vi "HardwareRangeStrings.vi"(8 "error in (no error)":errorcluster, 11 "Pstat IN":refnum<k7>) -> (0 "error out":errorcluster, 2 "Hardware Strings":T1={"I/E Ranges"=[], "First I/E Range"=0, "VchRanges"=[], "IchRanges"=[], "AchRanges"=[], "VchFilters"=[], "IchFilters"=[], "AchFilters"=[], "Family"="", "CA Speeds"=[], "ModelNo"=32} {"ModelNo" items=["PC4300"=32, "PC4750"=33, "PCI4300"=34, "PCI4750"=35, "FAS1"=16, "FC350"=17, "FAS2"=18, "FCI350"=19, "PC5600"=4, "PCI4G300"=36, "PCI4G750"=37, "FCIG350"=21, "REF3000"=5, "REF30K"=6]}, 3 "Pstat OUT":refnum<k7>)   [LabVIEW 2011]
panel:
  out "ModelNo":i32(ring)=32 items=["PC4300"=32, "PC4750"=33, "PCI4300"=34, "PCI4750"=35, "FAS1"=16, "FC350"=17, "FAS2"=18, "FCI350"=19, "PC5600"=4, "PCI4G300"=36, "PCI4G750"=37, "FCIG350"=21, "REF3000"=5, "REF30K"=6]
  out "TestIERange 100":i32
  out "TestIERange 0":i32
  out "CA Speeds":string[](array[string])=["Fast\n", "Normal", "Medium", "Slow"]
  out "Family":string="PC5"
  out "AchFilters":string[](array[string])=["30 mV", "300 mV", "3 V", "12 V"]
  out "IchFilters":string[](array[string])=["30 mV", "300 mV", "3 V", "12 V"]
  out "VchFilters":string[](array[string])=["30 mV", "300 mV", "3 V", "12 V"]
  out "AchRanges":string[](array[string])=["30 mV", "300 mV", "3 V", "12 V"]
  out "IchRanges":string[](array[string])=["30 mV", "300 mV", "3 V", "12 V"]
  out "VchRanges":string[](array[string])=["30 mV", "300 mV", "3 V", "12 V"]
  out "First I/E Range":i32=1
  out "I/E Ranges":string[](array[string])
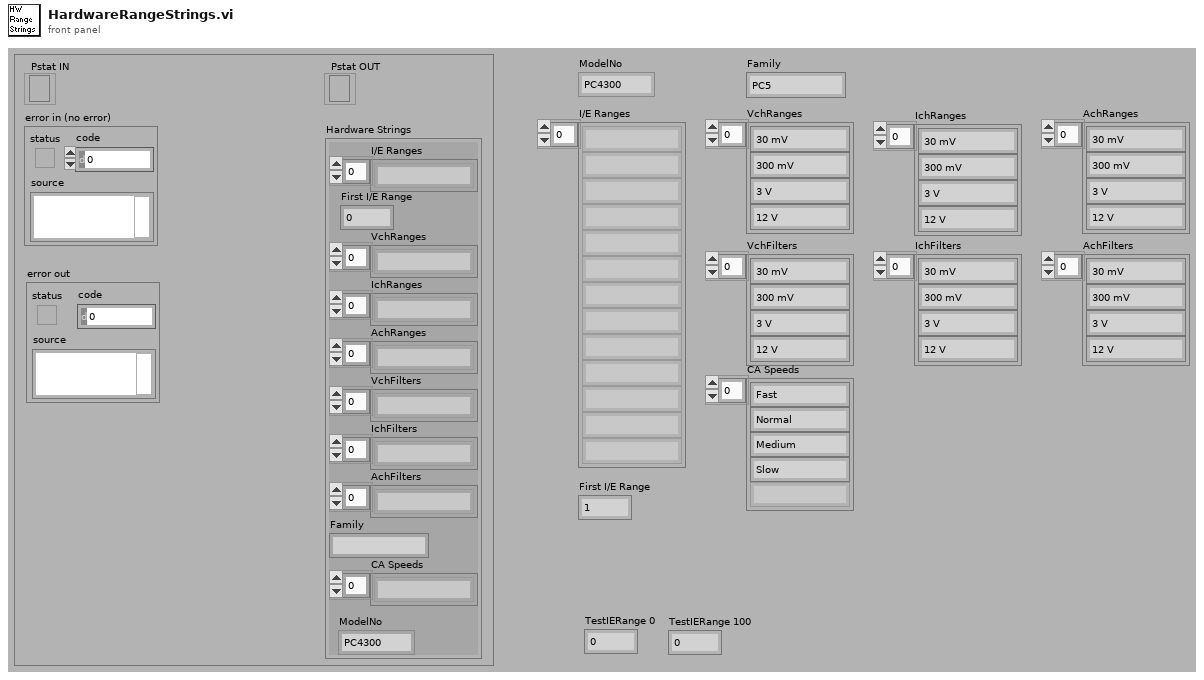
[diagram p1: front panel]
types:
  T1 = cluster{"I/E Ranges":string[], "First I/E Range":i32, "VchRanges":string[], "IchRanges":string[], "AchRanges":string[], "VchFilters":string[], "IchFilters":string[], "AchFilters":string[], "Family":string, "CA Speeds":string[], "ModelNo":i32}
  T2 = cluster{string[], i32, string[], string[], string[], string[], string[], string[], string, string[], "ModelNo":i32}
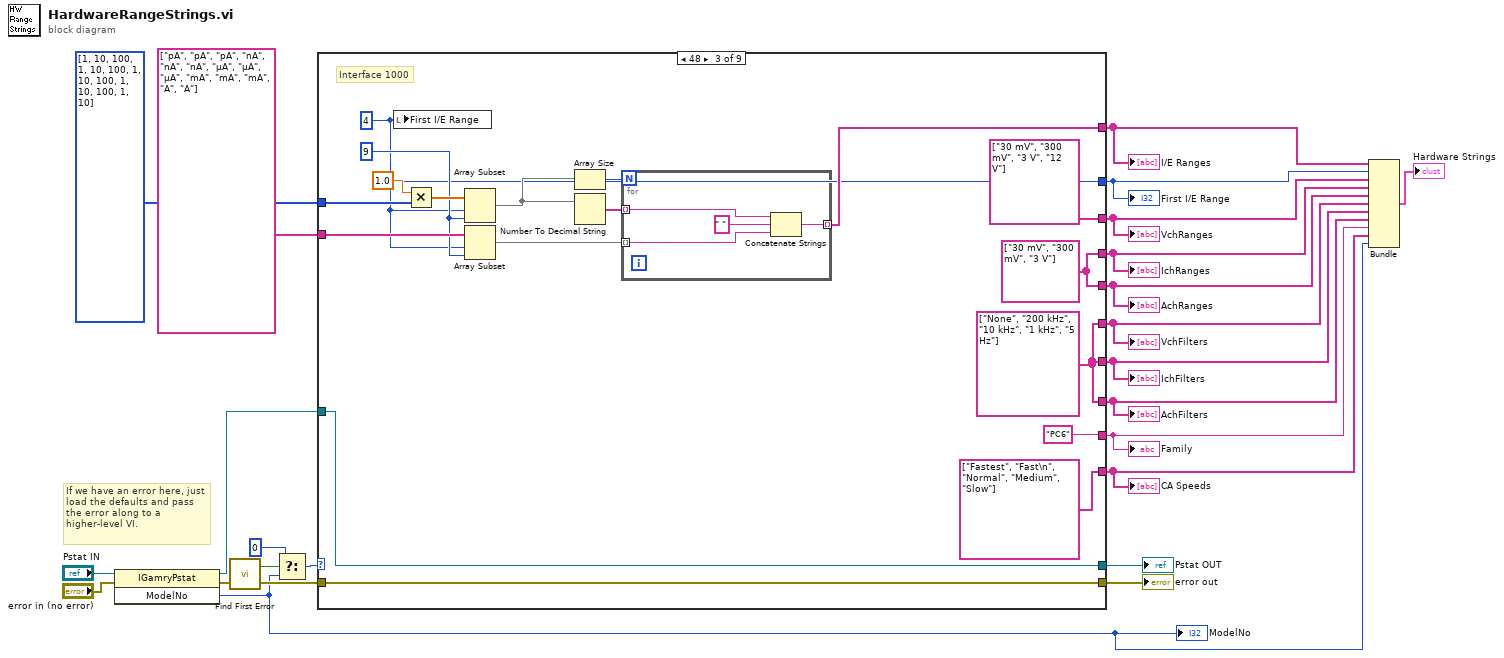
[diagram p0: block diagram]
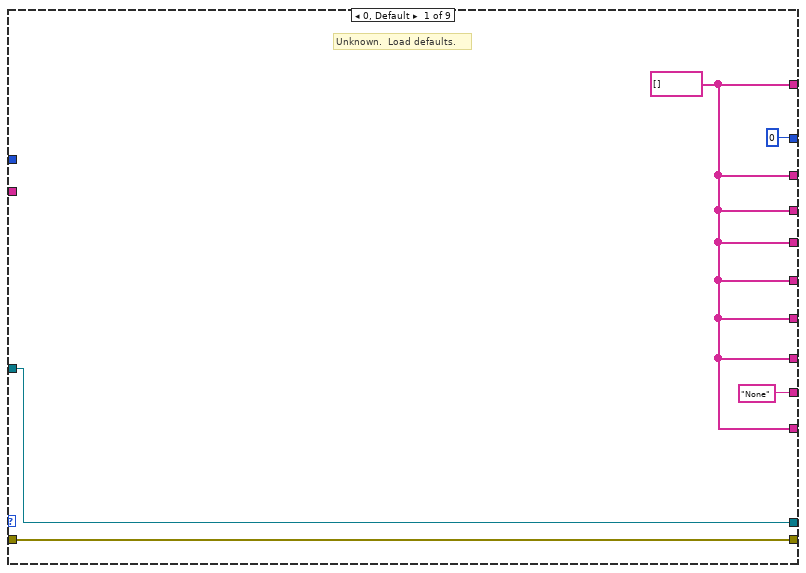
[diagram p2: hidden frame]
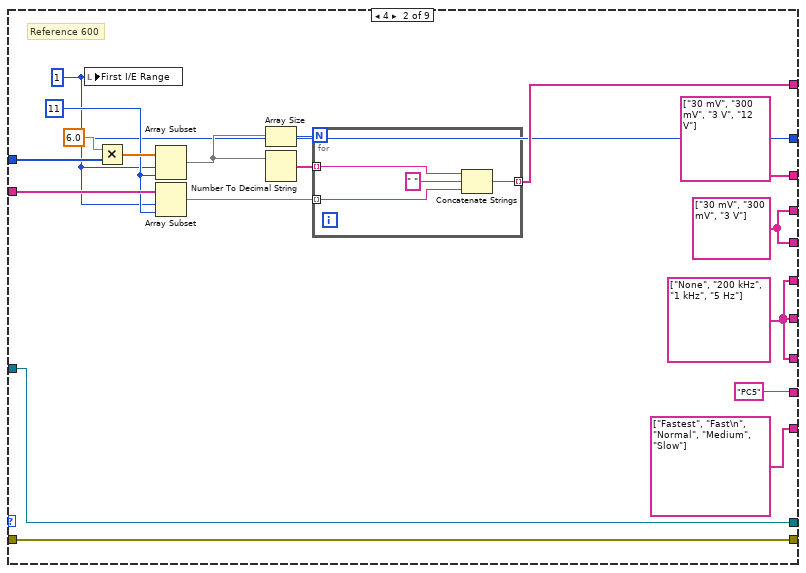
[diagram p3: hidden frame]
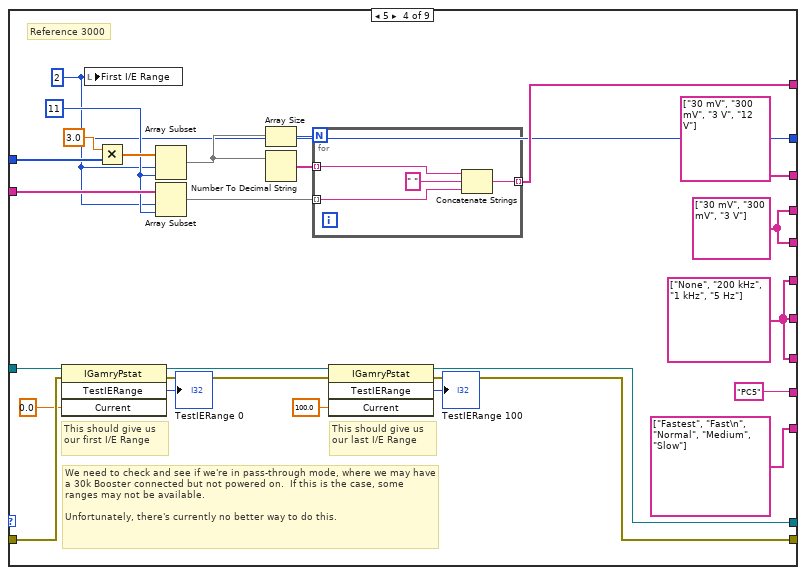
[diagram p4: hidden frame]
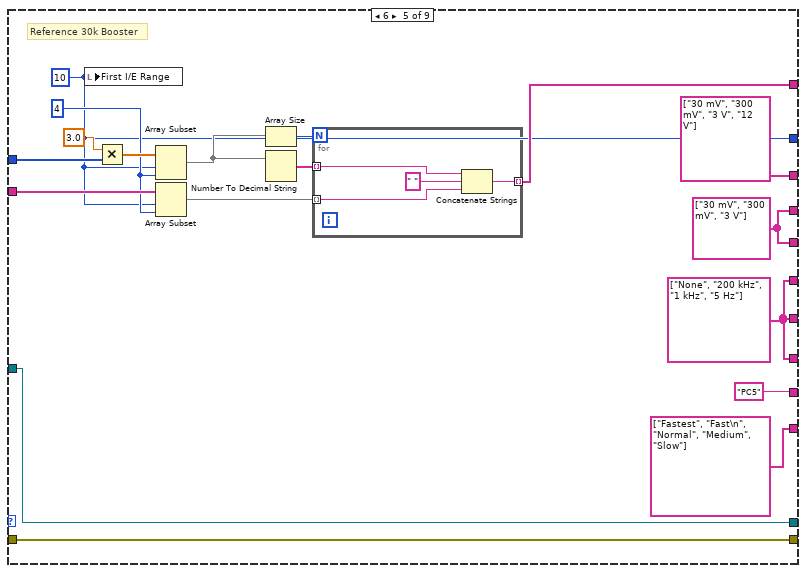
[diagram p5: hidden frame]
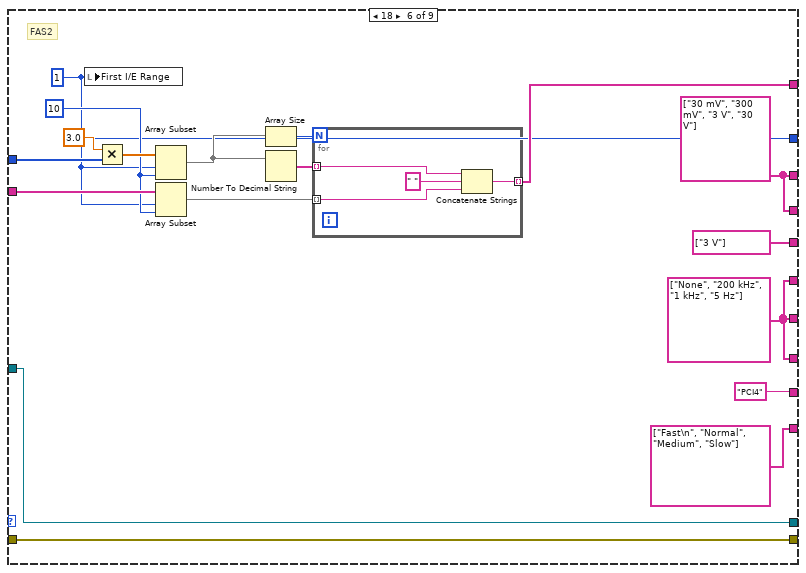
[diagram p6: hidden frame]
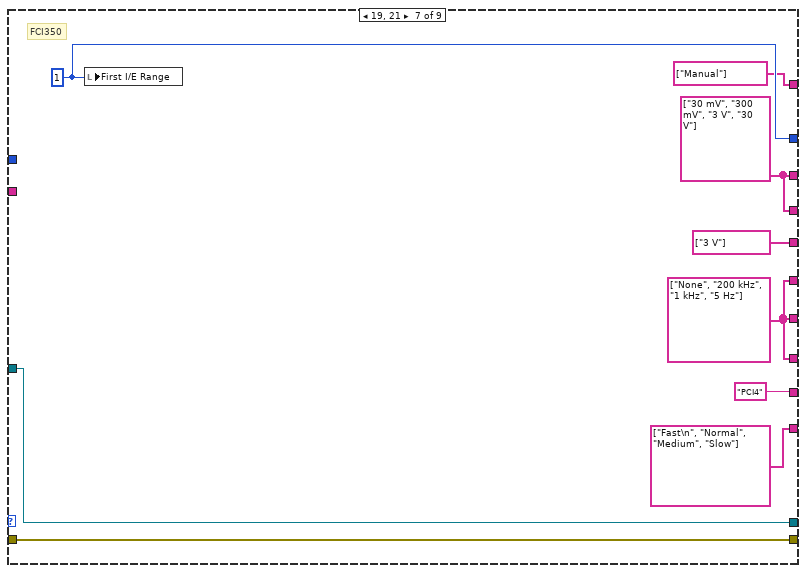
[diagram p7: hidden frame]
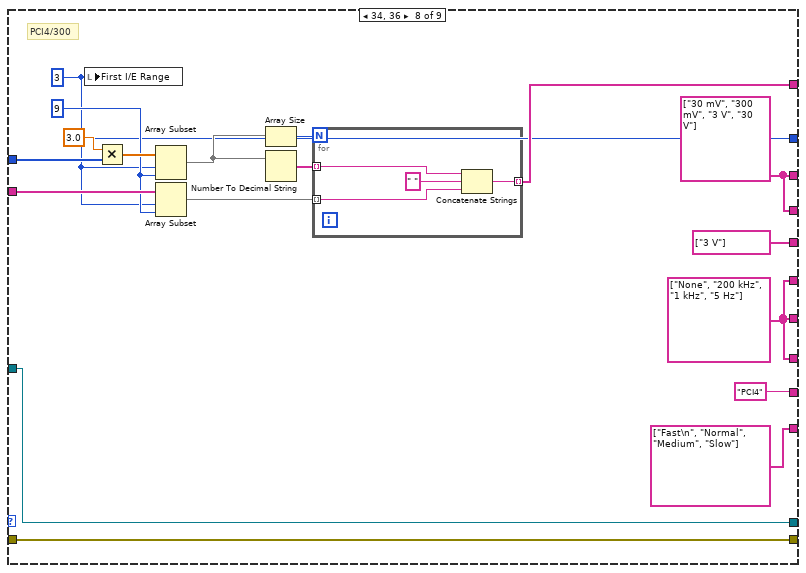
[diagram p8: hidden frame]
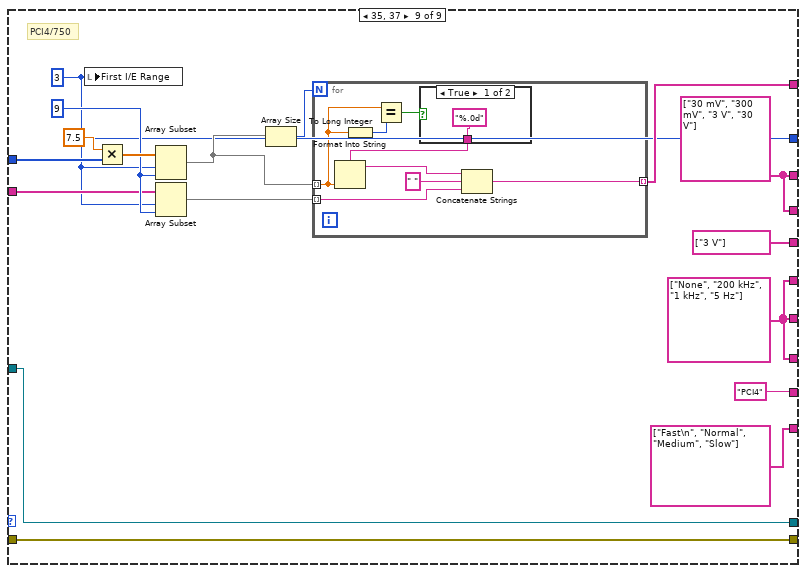
[diagram p9: hidden frame]
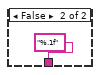
[diagram p10: hidden frame]
diagram:
  # "If we have an error here, just load the defaults and pass the error along to a higher-level VI."
  n1 = invoke class="IGamryPstat" method="ModelNo"(reference="Pstat IN", error in="error in (no error)") -> (reference out=w5:refnum<k7>, error out=w7:errorcluster, "ModelNo"=w2:i32)  [unwired: 1 in]
  "ModelNo" <- w2
  n2 = call <vilib>:"Find First Error.vi"("error in (no error)"=w7) -> ("error out"=w6:errorcluster, "error?"=w10:bool)  [unwired: 3 in]
  n3 = Select(t=0, s=w10, f=w2) -> (s? t:f=w9:i32)
  n4 = case shown="48" w9 {
    tunnel: i32[] [1, 10, 100, 1, 10, 100, 1, 10, 100, 1, 10, 100, 1, 10] -> [_ w43 w65 w95 w117 w139 _ w170 w183]
    tunnel: string[] ["pA", "pA", "pA", "nA", "nA", "nA", "µA", "µA", "µA", "mA", "mA", "mA", "A", "A"] -> [_ w45 w67 w97 w119 w141 _ w172 w184]
    tunnel: [w27 w38 w60 w90 w112 w134 string[] ["Manual"] w165 w182] -> w20
    tunnel: [0 w32 w54 w84 w106 w129 w152 w160 w181] -> w19
    tunnel: [w27 string[] ["30 mV", "300 mV", "3 V", "12 V"] string[] ["30 mV", "300 mV", "3 V", "12 V"] string[] ["30 mV", "300 mV", "3 V", "12 V"] string[] ["30 mV", "300 mV", "3 V", "12 V"] w128 w151 w159 w191] -> w18
    tunnel: [w27 w36 w58 w88 w110 w128 w151 w159 w191] -> w17
    tunnel: [w27 w36 w58 w88 w110 string[] ["3 V"] string[] ["3 V"] string[] ["3 V"] string[] ["3 V"]] -> w16
    tunnel: [w27 w35 w57 w87 w109 w132 w155 w163 w194] -> w15
    tunnel: [w27 w35 w57 w87 w109 w132 w155 w163 w194] -> w14
    tunnel: [w27 w35 w57 w87 w109 w132 w155 w163 w194] -> w13
    tunnel: ["None" "PC5" "PC6" "PC5" "PC5" "PCI4" "PCI4" "PCI4" "PCI4"] -> w12
    tunnel: [w27 string[] ["Fastest", "Fast\n", "Normal", "Medium", "Slow"] string[] ["Fastest", "Fast\n", "Normal", "Medium", "Slow"] string[] ["Fastest", "Fast\n", "Normal", "Medium", "Slow"] string[] ["Fastest", "Fast\n", "Normal", "Medium", "Slow"] string[] ["Fast\n", "Normal", "Medium", "Slow"] string[] ["Fast\n", "Normal", "Medium", "Slow"] string[] ["Fast\n", "Normal", "Medium", "Slow"] string[] ["Fast\n", "Normal", "Medium", "Slow"]] -> w11
    tunnel: w6 -> [w26 w31 w53 w82 w104 w127 w149 w158 w179]
    tunnel: w5 -> [w25 w30 w52 w83 w105 w126 w148 w157 w180]
    tunnel: [w26 w31 w53 w79 w104 w127 w149 w158 w179] -> w4
    tunnel: [w25 w30 w52 w77 w105 w126 w148 w157 w180] -> w3
    frame 0, Default {
      w27 = string[] []
      # "Unknown.  Load defaults."
    }
    frame 4 {
      w35 = string[] ["None", "200 kHz", "1 kHz", "5 Hz"]
      w36 = string[] ["30 mV", "300 mV", "3 V"]
      w32 = 1
      w39 = 11 ("length")
      # "Reference 600"
      n5 = local write "First I/E Range"(w32) -> ()
      n6 = Multiply(x=sgl 6.0, y=w43) -> (x*y=w46:sgl[])
      n7 = Array Subset(array=w46, index=w32, length=w39) -> (w42:sgl[])
      n8 = Array Subset(array=w45, index=w32, length=w39) -> (w41:string[])
      n9 = Array Size(array=w42) -> (size(s)=w44:i32)
      n10 = Number To Decimal String(number=w42) -> (decimal integer string=w40:string[])  [unwired: 1 in]
      n11 = for {
        N: w44 -> [_]
        tunnel: w41 -> [w50] mode=indexing
        tunnel: w40 -> [w49] mode=indexing
        tunnel: [w48] -> w38 mode=indexing
        n12 = Concatenate Strings(w49, " " ("string"), w50) -> (w48:string)
      }
    }
    frame 48 {
      w57 = string[] ["None", "200 kHz", "10 kHz", "1 kHz", "5 Hz"]
      w58 = string[] ["30 mV", "300 mV", "3 V"]
      w54 = 4
      w61 = 9 ("length")
      # "Interface 1000"
      n13 = local write "First I/E Range"(w54) -> ()
      n14 = Multiply(x=sgl 1.0, y=w65) -> (x*y=w68:sgl[])
      n15 = Array Subset(array=w68, index=w54, length=w61) -> (w64:sgl[])
      n16 = Array Subset(array=w67, index=w54, length=w61) -> (w63:string[])
      n17 = Array Size(array=w64) -> (size(s)=w66:i32)
      n18 = Number To Decimal String(number=w64) -> (decimal integer string=w62:string[])  [unwired: 1 in]
      n19 = for {
        N: w66 -> [_]
        tunnel: w63 -> [w72] mode=indexing
        tunnel: w62 -> [w71] mode=indexing
        tunnel: [w70] -> w60 mode=indexing
        n20 = Concatenate Strings(w71, " " ("string"), w72) -> (w70:string)
      }
    }
    frame 5 {
      w87 = string[] ["None", "200 kHz", "1 kHz", "5 Hz"]
      w88 = string[] ["30 mV", "300 mV", "3 V"]
      w84 = 2
      w91 = 11 ("length")
      # "This should give us our last I/E Range"
      # "This should give us our first I/E Range"
      # "We need to check and see if we're in pass-through mode, where we may have a 30k Booster connected but not powered on.  If this is the case, some ranges may not be available.\n\nUnfortunately, there's currently no better way to do this."
      # "Reference 3000"
      n21 = invoke class="IGamryPstat" method="TestIERange"(reference=w83, error in=w82, "Current"=sgl 0.0) -> (reference out=w78:refnum<k7>, error out=w80:errorcluster, "TestIERange"=→"TestIERange 0":i32)  [unwired: 1 in, 1 out]
      n22 = local write "First I/E Range"(w84) -> ()
      n23 = Multiply(x=sgl 3.0, y=w95) -> (x*y=w98:sgl[])
      n24 = Array Subset(array=w98, index=w84, length=w91) -> (w94:sgl[])
      n25 = Array Subset(array=w97, index=w84, length=w91) -> (w93:string[])
      n26 = Array Size(array=w94) -> (size(s)=w96:i32)
      n27 = Number To Decimal String(number=w94) -> (decimal integer string=w92:string[])  [unwired: 1 in]
      n28 = for {
        N: w96 -> [_]
        tunnel: w93 -> [w102] mode=indexing
        tunnel: w92 -> [w101] mode=indexing
        tunnel: [w100] -> w90 mode=indexing
        n29 = Concatenate Strings(w101, " " ("string"), w102) -> (w100:string)
      }
      n30 = invoke class="IGamryPstat" method="TestIERange"(reference=w78, error in=w80, "Current"=sgl 100.0) -> (reference out=w77:refnum<k7>, error out=w79:errorcluster, "TestIERange"=→"TestIERange 100":i32)  [unwired: 1 in, 1 out]
    }
    frame 6 {
      w109 = string[] ["None", "200 kHz", "1 kHz", "5 Hz"]
      w110 = string[] ["30 mV", "300 mV", "3 V"]
      w106 = 10
      w113 = 4 ("length")
      # "Reference 30k Booster"
      n31 = local write "First I/E Range"(w106) -> ()
      n32 = Multiply(x=sgl 3.0, y=w117) -> (x*y=w120:sgl[])
      n33 = Array Subset(array=w120, index=w106, length=w113) -> (w116:sgl[])
      n34 = Array Subset(array=w119, index=w106, length=w113) -> (w115:string[])
      n35 = Array Size(array=w116) -> (size(s)=w118:i32)
      n36 = Number To Decimal String(number=w116) -> (decimal integer string=w114:string[])  [unwired: 1 in]
      n37 = for {
        N: w118 -> [_]
        tunnel: w115 -> [w124] mode=indexing
        tunnel: w114 -> [w123] mode=indexing
        tunnel: [w122] -> w112 mode=indexing
        n38 = Concatenate Strings(w123, " " ("string"), w124) -> (w122:string)
      }
    }
    frame 18 {
      w132 = string[] ["None", "200 kHz", "1 kHz", "5 Hz"]
      w128 = string[] ["30 mV", "300 mV", "3 V", "30 V"]
      w129 = 1
      w135 = 10 ("length")
      # "FAS2"
      n39 = local write "First I/E Range"(w129) -> ()
      n40 = Multiply(x=sgl 3.0, y=w139) -> (x*y=w142:sgl[])
      n41 = Array Subset(array=w142, index=w129, length=w135) -> (w138:sgl[])
      n42 = Array Subset(array=w141, index=w129, length=w135) -> (w137:string[])
      n43 = Array Size(array=w138) -> (size(s)=w140:i32)
      n44 = Number To Decimal String(number=w138) -> (decimal integer string=w136:string[])  [unwired: 1 in]
      n45 = for {
        N: w140 -> [_]
        tunnel: w137 -> [w146] mode=indexing
        tunnel: w136 -> [w145] mode=indexing
        tunnel: [w144] -> w134 mode=indexing
        n46 = Concatenate Strings(w145, " " ("string"), w146) -> (w144:string)
      }
    }
    frame 19, 21 {
      w155 = string[] ["None", "200 kHz", "1 kHz", "5 Hz"]
      w151 = string[] ["30 mV", "300 mV", "3 V", "30 V"]
      w152 = 1
      # "FCI350"
      n47 = local write "First I/E Range"(w152) -> ()
    }
    frame 34, 36 {
      w163 = string[] ["None", "200 kHz", "1 kHz", "5 Hz"]
      w159 = string[] ["30 mV", "300 mV", "3 V", "30 V"]
      w160 = 3
      w166 = 9 ("length")
      # "PCI4/300"
      n48 = local write "First I/E Range"(w160) -> ()
      n49 = Multiply(x=sgl 3.0, y=w170) -> (x*y=w173:sgl[])
      n50 = Array Subset(array=w173, index=w160, length=w166) -> (w169:sgl[])
      n51 = Array Subset(array=w172, index=w160, length=w166) -> (w168:string[])
      n52 = Array Size(array=w169) -> (size(s)=w171:i32)
      n53 = Number To Decimal String(number=w169) -> (decimal integer string=w167:string[])  [unwired: 1 in]
      n54 = for {
        N: w171 -> [_]
        tunnel: w168 -> [w177] mode=indexing
        tunnel: w167 -> [w176] mode=indexing
        tunnel: [w175] -> w165 mode=indexing
        n55 = Concatenate Strings(w176, " " ("string"), w177) -> (w175:string)
      }
    }
    frame 35, 37 {
      w181 = 3
      w186 = 9 ("length")
      w194 = string[] ["None", "200 kHz", "1 kHz", "5 Hz"]
      w191 = string[] ["30 mV", "300 mV", "3 V", "30 V"]
      # "PCI4/750"
      n56 = local write "First I/E Range"(w181) -> ()
      n57 = Multiply(x=sgl 7.5, y=w183) -> (x*y=w189:sgl[])
      n58 = Array Subset(array=w189, index=w181, length=w186) -> (w185:sgl[])
      n59 = Array Subset(array=w184, index=w181, length=w186) -> (w187:string[])
      n60 = Array Size(array=w185) -> (size(s)=w188:i32)
      n61 = for {
        N: w188 -> [_]
        tunnel: w187 -> [w202] mode=indexing
        tunnel: [w201] -> w182 mode=indexing
        tunnel: w185 -> [w198] mode=indexing
        n62 = To Long Integer(number=w198) -> (32bit integer=w199:i32)
        n63 = Equal?(x=w198, y=w199) -> (x = y?=w197:bool)
        n64 = case shown="True" w197 {
          tunnel: ["%.0d" ("format string") "%.1f" ("format string")] -> w196
          frame True {
          }
          frame False {
          }
        }
        n65 = Format Into String(format string=w196, w198) -> (resulting string=w200:string)  [unwired: 2 in, 1 out]
        n66 = Concatenate Strings(w200, " " ("string"), w202) -> (w201:string)
      }
    }
  }
  "I/E Ranges" <- w20
  "First I/E Range" <- w19
  "VchRanges" <- w18
  "IchRanges" <- w17
  "AchRanges" <- w16
  "VchFilters" <- w15
  "IchFilters" <- w14
  "AchFilters" <- w13
  "Family" <- w12
  "CA Speeds" <- w11
  "error out" <- w4
  "Pstat OUT" <- w3
  n67 = Bundle(w20, w19, w18, w17, w16, w15, w14, w13, w12, w11, "ModelNo"=w2) -> (→"Hardware Strings":T2)  [unwired: 1 in]
